vi "Read Export Build Specification.vi"(8 "error in (no error)":errorcluster, 11 "Export in":refnum<class "Export.lvclass">) -> (0 "error out":errorcluster, 2 "Export Build Specification":path, 3 "Export out":refnum<class "Export.lvclass">)   [LabVIEW 2017, in "CL_G3_VIComponentBuilder.lvlib" / "Export.lvclass"]
uses:
  Export.lvclass
  Export.lvclass/Export.ctl
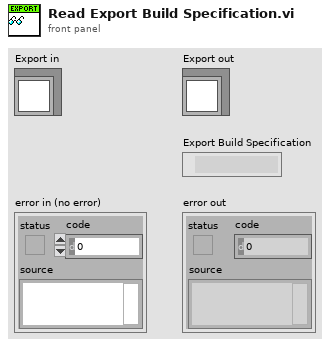
[diagram p1: front panel]
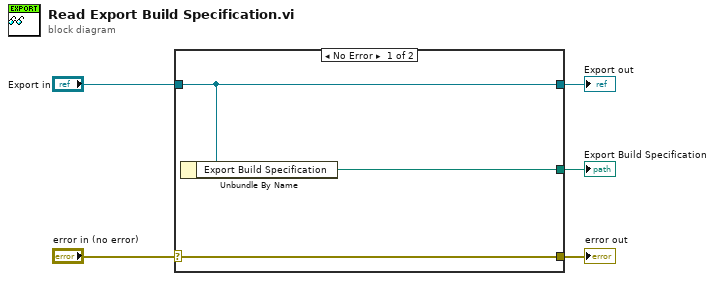
[diagram p0: block diagram]
diagram:
  n1 = case shown="No Error" "error in (no error)" {
    selector: "error in (no error)" -> [w8 w9]
    tunnel: [w8 w9] -> w4
    tunnel: [w7 w10] -> w2
    tunnel: "Export in" -> [w7 w10]
    tunnel: [w6 _] -> w1
    frame No Error {
      n2 = Unbundle By Name(w7) -> ("Export Build Specification"=w6:path)
    }
    frame Error {
    }
  }
  "error out" <- w4
  "Export out" <- w2
  "Export Build Specification" <- w1
